vi "FPGA_DMAReadFromStream.vi"(8 "error in (no error)":errorcluster, 9 "Timeout (ms)":i32=5000, 10 "NumberOfElements":u32, 11 "DMADevRef In":T1) -> (0 "error out":errorcluster, 1 "Elements Remaining":u32, 2 "Data":u32[](array[numeric]), 3 "DMADevRef Out":T1, 4 "Timed Out":bool)   [LabVIEW 2017]
uses:
  <vilib>/Rock Robotics/SystemInterfaces/DMA/FPGA_DMADevRef.ctl
  <vilib>/Rock Robotics/SystemInterfaces/System/FPGA_SystemFPGA Ref Global.vi
  <vilib>/Utility/error.llb/Error Cluster From Error Code.vi
  <vilib>/rvi/errors/niLvFpgaAdjustHostInterfaceError.vi
  <vilib>/rvi/interface/nirviMethod/nirviMethod.xnode
  <vilib>/Rock Robotics/SystemInterfaces/System/FPGA_SystemFRC FPGA Ref.ctl
  <vilib>/FPGAPlugInAG/Dynamic/niLvFpga_ReadFifo_Dynamic.vi
  <vilib>/rvi/errors/niLvFpgaMergeErrorWithErrorCode.vi
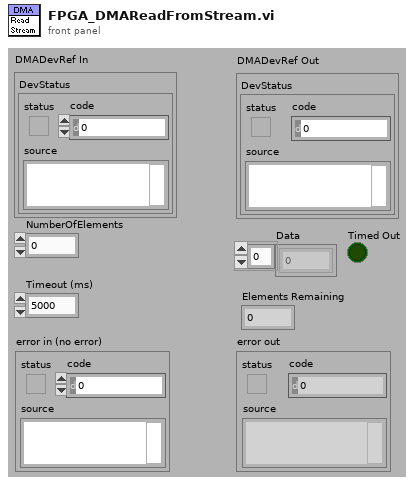
[diagram p1: front panel]
types:
  T1 = typedef "FPGA_DMADevRef.ctl" = cluster{"DevStatus":errorcluster}
  T2 = typedef "FPGA_SystemFRC FPGA Ref.ctl" = refnum<k20>
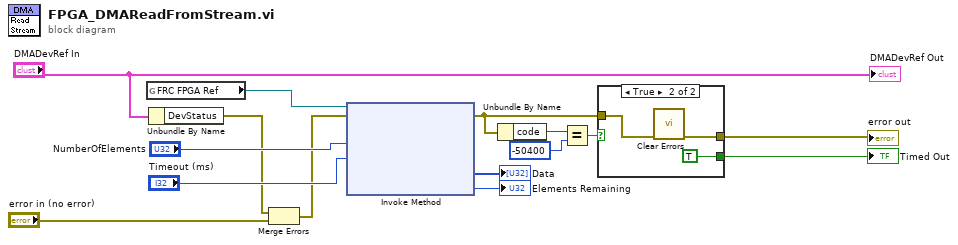
[diagram p0: block diagram]
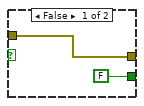
[diagram p2: hidden frame]
diagram:
  n1 = global read "FPGA_SystemFPGA Ref Global.vi" "FRC FPGA Ref"() -> (w4:T2)
  n2 = Unbundle By Name("DMADevRef In") -> ("DevStatus"=w3:errorcluster)
  n3 = Merge Errors(w3, "error in (no error)") -> (w2:errorcluster)
  n4 = xnode "Invoke Method"("FPGA VI Reference In"=w4, "error in"=w2, "Number of Elements"="NumberOfElements", "Timeout (ms)"="Timeout (ms)") -> ("error out"=w5:errorcluster, "Data"=→"Data":u32[], "Elements Remaining"=→"Elements Remaining":u32)  [unwired: 1 out]
  n5 = Unbundle By Name(w5) -> ("code"=w7:i32)
  n6 = Equal?(x=w7, y=-50400 ("code")) -> (x = y?=w6:bool)
  n7 = case shown="True" w6 {
    tunnel: w5 -> [w17 w20]
    tunnel: [w17 w19] -> w14
    tunnel: [FALSE TRUE] -> w13
    frame False {
    }
    frame True {
      n8 = call <vilib>:"Clear Errors.vi"("error in (no error)"=w20) -> ("error out"=w19:errorcluster)  [unwired: 1 in, 5 out]
    }
  }
  "error out" <- w14
  "Timed Out" <- w13
  "DMADevRef Out" <- "DMADevRef In"
